vi "setup.vi"(0 "PicamModel":T1=715 items=["---PIXIS 100 SERIES---"=1000, "PixisSeries"=0, "Pixis100BR"=5, "---PI-MAX4 SERIES---"=1001, "Pimax4Series"=700, "PiMax41024EM"=715]) -> (7 "camera handle":u64, 10 "error out":errorcluster)   [LabVIEW 2019, in "PICam.lvlib"]
uses:
  PICam.lvlib
  types/PicamModel.ctl
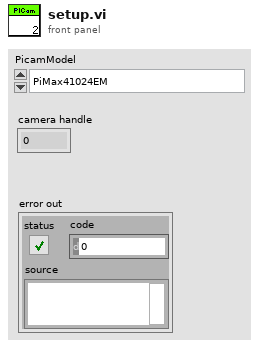
[diagram p1: front panel]
types:
  T1 = typedef "PicamModel.ctl" = u32
  T2 = typedef "PICam.lvlib/PicamCameraID.ctl" = cluster{"PicamModel":T3, "PicamComputerInterface":T4, "sensor_name":T5, "serial_number":T6}
  T3 = typedef "PICAM.lvlib/PicamModel.ctl" = u32
  T4 = typedef "PICAM.lvlib/PicamComputerInterface.ctl" = u32
  T5 = typedef "PICAM.lvlib/sensor_name.ctl" = cluster{"U8":u8, "U8 2":u8, "U8 3":u8, "U8 4":u8, "U8 5":u8, "U8 6":u8, "U8 7":u8, "U8 8":u8, "U8 9":u8, "U8 10":u8, "U8 11":u8, "U8 12":u8, "U8 13":u8, "U8 14":u8, "U8 15":u8, "U8 16":u8, "U8 17":u8, "U8 18":u8, "U8 19":u8, "U8 20":u8, "U8 21":u8, "U8 22":u8, "U8 23":u8, "U8 24":u8, "U8 25":u8, "U8 26":u8, "U8 27":u8, "U8 28":u8, "U8 29":u8, "U8 30":u8, "U8 31":u8, "U8 32":u8, "U8 33":u8, "U8 34":u8, "U8 35":u8, "U8 36":u8, "U8 37":u8, "U8 38":u8, "U8 39":u8, "U8 40":u8, "U8 41":u8, "U8 42":u8, "U8 43":u8, "U8 44":u8, "U8 45":u8, "U8 46":u8, "U8 47":u8, "U8 48":u8, "U8 49":u8, "U8 50":u8, "U8 51":u8, "U8 52":u8, "U8 53":u8, "U8 54":u8, "U8 55":u8, "U8 56":u8, "U8 57":u8, "U8 58":u8, "U8 59":u8, "U8 60":u8, "U8 61":u8, "U8 62":u8, "U8 63":u8, "U8 64":u8}
  T6 = typedef "PICAM.lvlib/serial_number.ctl" = cluster{"U8":u8, "U8 2":u8, "U8 3":u8, "U8 4":u8, "U8 5":u8, "U8 6":u8, "U8 7":u8, "U8 8":u8, "U8 9":u8, "U8 10":u8, "U8 11":u8, "U8 12":u8, "U8 13":u8, "U8 14":u8, "U8 15":u8, "U8 16":u8, "U8 17":u8, "U8 18":u8, "U8 19":u8, "U8 20":u8, "U8 21":u8, "U8 22":u8, "U8 23":u8, "U8 24":u8, "U8 25":u8, "U8 26":u8, "U8 27":u8, "U8 28":u8, "U8 29":u8, "U8 30":u8, "U8 31":u8, "U8 32":u8, "U8 33":u8, "U8 34":u8, "U8 35":u8, "U8 36":u8, "U8 37":u8, "U8 38":u8, "U8 39":u8, "U8 40":u8, "U8 41":u8, "U8 42":u8, "U8 43":u8, "U8 44":u8, "U8 45":u8, "U8 46":u8, "U8 47":u8, "U8 48":u8, "U8 49":u8, "U8 50":u8, "U8 51":u8, "U8 52":u8, "U8 53":u8, "U8 54":u8, "U8 55":u8, "U8 56":u8, "U8 57":u8, "U8 58":u8, "U8 59":u8, "U8 60":u8, "U8 61":u8, "U8 62":u8, "U8 63":u8, "U8 64":u8}
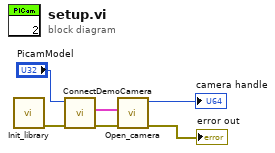
[diagram p0: block diagram]
diagram:
  n1 = call "Init_library.vi"() -> ("error out"=w6:errorcluster)  [unwired: 11 in]
  n2 = call "ConnectDemoCamera.vi"("error in"=w6, "PicamModel"="PicamModel") -> ("error out"=w4:errorcluster, "PicamCameraID"=w3:T2)  [unwired: 8 in]
  n3 = call "Open_camera.vi"("error in"=w4, "PicamCameraID"=w3) -> ("error out"=→"error out":errorcluster, "camera handler out"=→"camera handle":u64)  [unwired: 8 in]
